vi "Initialize Instrument.vi"(8 "error in (no error)":errorcluster, 10 "Reset":bool, 11 "U2000 in":refnum<class "U2000.lvclass">) -> (0 "error out":errorcluster, 3 "U2000 out":refnum<class "U2000.lvclass">)   [LabVIEW 2020, in "U2000.lvclass"]
uses:
  U2000.lvclass
  C:/Sandbox/Git_Sandbox/WiSpry Test Framework source code (LV20)/WiSpry Test Framework/Instruments/Instrument.lvclass
  Instrument.lvclass/Instrument.ctl
  <instrlib>/Agilent U2000 Series/Public/Data/Low Level/Initiate (Continuous).vi
  Instrument.lvclass
  <instrlib>/Agilent U2000 Series/Agilent U2000 Series.lvlib
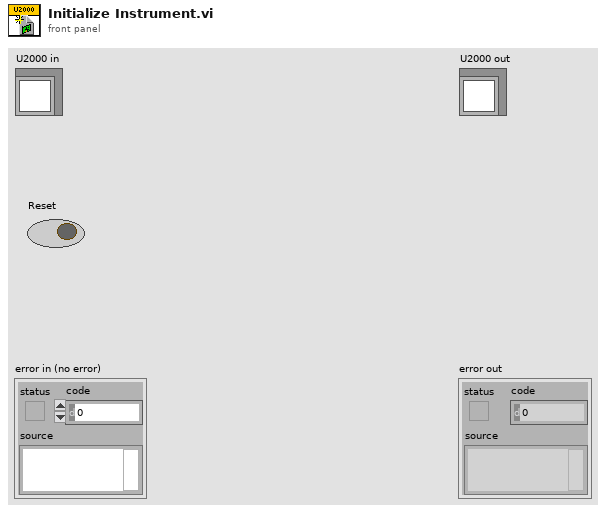
[diagram p1: front panel]
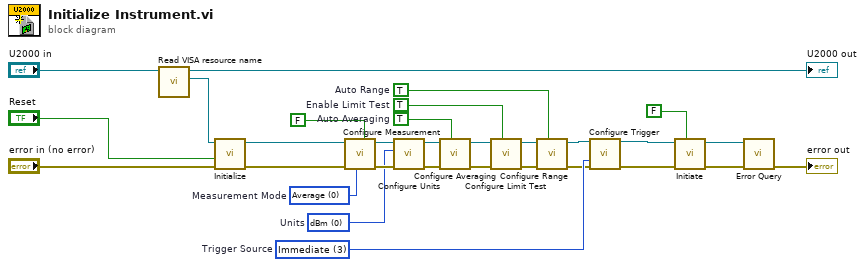
[diagram p0: block diagram]
diagram:
  w10 = 0 items=["dBm", "Watts"]  # Units
  w22 = 3 items=["Bus", "External", "Hold", "Immediate", "Internal A"]  # Trigger Source
  w23 = 0 items=["Average", "Normal"]  # Measurement Mode
  w15 = TRUE  # Enable Limit Test
  w16 = TRUE  # Auto Averaging
  w14 = TRUE  # Auto Range
  n1 = call "Read VISA resource name.vi"("Instrument in"="U2000 in") -> ("VISA resource name"=w26:refnum<visa-resource-name>, "Instrument out"=→"U2000 out":refnum<class "U2000.lvclass">)  [unwired: 9 in]
  n2 = call <instrlib>:"Initialize.vi"("error in (no error)"="error in (no error)", "Reset (True)"="Reset", "VISA resource name"=w26) -> ("error out"=w5:errorcluster, "VISA resource name out"=w4:refnum<visa-resource-name>)  [unwired: 7 in]
  n3 = call <instrlib>:"Configure Measurement.vi"("Enable Gate Feed (T: Enable)"=FALSE, "Measurement Function (0: Average)"=w23, "error in (no error)"=w5, "VISA resource name"=w4) -> ("error out"=w24:errorcluster, "VISA resource name out"=w25:refnum<visa-resource-name>)  [unwired: 6 in]
  n4 = call <instrlib>:"Configure Units.vi"("error in (no error)"=w24, "Units (0: dBm)"=w10, "VISA resource name"=w25) -> ("error out"=w19:errorcluster, "VISA resource name out"=w20:refnum<visa-resource-name>)  [unwired: 1 in, 6 out]
  n5 = call <instrlib>:"Configure Averaging.vi"("Enable Averaging (T: Enable)"=w16, "error in (no error)"=w19, "VISA resource name"=w20) -> ("error out"=w17:errorcluster, "VISA resource name out"=w18:refnum<visa-resource-name>)  [unwired: 7 in]
  n6 = call <instrlib>:"Configure Limit Test.vi"("Limit Test (T: Enable)"=w15, "error in (no error)"=w17, "VISA resource name"=w18) -> ("error out"=w12:errorcluster, "VISA resource name out"=w13:refnum<visa-resource-name>)  [unwired: 2 in, 5 out]
  n7 = call <instrlib>:"Configure Range.vi"("Auto Range (T: Enable)"=w14, "error in (no error)"=w12, "VISA resource name"=w13) -> ("error out"=w11:errorcluster, "VISA resource name out"=w21:refnum<visa-resource-name>)  [unwired: 7 in]
  n8 = call <instrlib>:"Configure Trigger.vi"("VISA resource name"=w21, "Trigger Source (3: Immediate)"=w22, "error in (no error)"=w11) -> ("VISA resource name out"=w8:refnum<visa-resource-name>, "error out"=w9:errorcluster)  [unwired: 5 in, 6 out]
  n9 = call-poly <instrlib>:"Initiate.vi"("Enable Initiate Continuous (T: Enable)"=FALSE ("Continuous mode"), "error in (no error)"=w9, "VISA resource name"=w8) -> ("error out"=w2:errorcluster, "VISA resource name out"=w3:refnum<visa-resource-name>)  [unwired: 7 in]
  n10 = call <instrlib>:"Error Query.vi"("error in (no error)"=w2, "VISA resource name"=w3) -> ("error out"=→"error out":errorcluster)  [unwired: 6 in, 3 out]
